vi "Build Do.vi"(5 "Target":refnum<vi>, 6 "Class Name":string, 7 "AppInst":refnum<vi>, 8 "error in (no error)":errorcluster, 9 "Actor class path":path, 10 "Do Method path":path, 11 "Target Method path":path) -> (0 "error out":errorcluster)   [LabVIEW 2020, in "Message Maker.lvlib"]
uses:
  Message Maker.lvlib
  <vilib>/Utility/traverseref.llb/TRef TravTarget.ctl
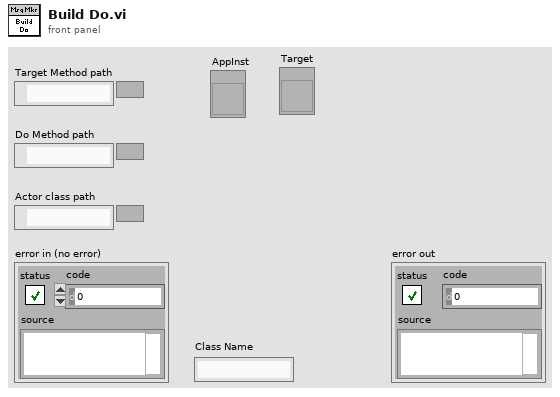
[diagram p1: front panel]
types:
  T1 = enum32{"Invalid", "Standard", "Closed", "Hidden", "Minimized", "Maximized"}
  T2 = typedef "TRef TravTarget.ctl" = enum16{"FP", "BD", "Other"}
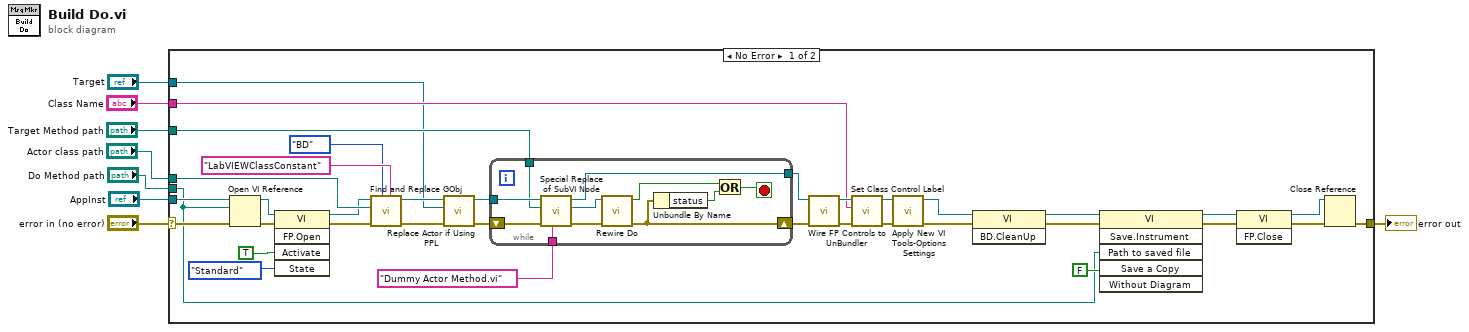
[diagram p0: block diagram]
diagram:
  n1 = case shown="No Error" "error in (no error)" {
    selector: "error in (no error)" -> [w32 w56]
    tunnel: [w42 w56] -> w8
    tunnel: "Target Method path" -> [w30 _]
    tunnel: "Do Method path" -> [w23 _]
    tunnel: "Actor class path" -> [w33 _]
    tunnel: "Class Name" -> [w31 _]
    tunnel: "AppInst" -> [w24 _]
    tunnel: "Target" -> [w10 _]
    frame No Error {
      n2 = Open VI Reference(application reference (local)=w24, vi path=w23, error in (no error)=w32) -> (vi reference=w26:refnum<vi>, error out=w25:errorcluster)  [unwired: 3 in]
      n3 = invoke class="VI" method="FP.Open"(reference=w26, error in=w25, "Activate"=TRUE ("Activate?"), "State"=T1."Standard") -> (reference out=w14:refnum<vi>, error out=w13:errorcluster)  [unwired: 1 in, 3 out]
      n4 = call "Find and Replace GObj.vi"("GObj Class Name"="LabVIEWClassConstant" ("Class Name"), "Traverse Target"=TRef_TravTarget."BD", "error in (no error)"=w13, "Class Path"=w33, "vi reference in"=w14) -> ("error out"=w11:errorcluster, "vi reference out"=w16:refnum<vi>)  [unwired: 4 in, 1 out]
      n5 = call "Replace Actor if Using PPL.vi"("error in (no error)"=w11, "Target"=w10, "Send VI ref in"=w16) -> ("error out"=w17:errorcluster, "Send VI ref out"=w15:refnum<vi>)  [unwired: 7 in]
      n6 = while {
        tunnel: w15 -> [w55]
        tunnel: w30 -> [w53]
        tunnel: [w51] -> w18
        shift-right: [w49] -> w12
        shift-left: w17 -> [w54]
        tunnel: "Dummy Actor Method.vi" -> [w45]
        stop <- w46 stop-if-true
        n7 = call "Special Replace of SubVI Node.vi"("GObj Label"=w45, "error in (no error)"=w54, "Class Path"=w53, "vi reference in"=w55) -> ("error out"=w52:errorcluster, "Replace"=w50:refnum<vi>, "vi reference out"=w51:refnum<vi>)  [unwired: 5 in]
        n8 = call "Rewire Do.vi"("error in (no error)"=w52, "Replace"=w50) -> ("error out"=w49:errorcluster, "done?"=w47:bool)  [unwired: 8 in]
        n9 = Unbundle By Name(w49) -> ("status"=w48:bool)
        n10 = Or(x=w47, y=w48) -> (x .or. y?=w46:bool)
      }
      n11 = call "Wire FP Controls to UnBundler.vi"("error in (no error)"=w12, "vi reference in"=w18) -> ("error out"=w35:errorcluster, "vi reference out"=w34:refnum<vi>)  [unwired: 8 in]
      n12 = call "Set Class Control Label.vi"("error in (no error)"=w35, "Class Name"=w31, "vi reference in"=w34) -> ("error out"=w19:errorcluster, "vi reference out"=w22:refnum<vi>)  [unwired: 7 in]
      n13 = call <vilib>:"Apply New VI Tools-Options Settings.vi"("error in (no error)"=w19, "VI Refnum"=w22) -> ("error out"=w20:errorcluster, "dup VI Refnum"=w21:refnum<vi>)  [unwired: 8 in]
      n14 = invoke class="VI" method="BD.CleanUp"(reference=w21, error in=w20) -> (reference out=w28:refnum<vi>, error out=w27:errorcluster)  [unwired: 1 in, 1 out]
      n15 = invoke class="VI" method="Save.Instrument"(reference=w28, error in=w27, "Path to saved file"=w23, "Save a Copy"=FALSE) -> (reference out=w38:refnum<vi>, error out=w39:errorcluster)  [unwired: 2 in, 4 out]
      n16 = invoke class="VI" method="FP.Close"(reference=w38, error in=w39) -> (reference out=w36:refnum<vi>, error out=w37:errorcluster)  [unwired: 1 in, 1 out]
      n17 = Close Reference(reference=w36, error in (no error)=w37) -> (error out=w42:errorcluster)
    }
    frame Error {
    }
  }
  "error out" <- w8
